vi "Append Rx Map Value to String.vi"(10 "value":T1, 11 "initial string":string) -> (3 "resulting string":string)   [LabVIEW 2020]
uses:
  Git/niveristand-ballard-milStd1553-custom-device/Source/Custom Device Support/Engine/Implementation/Rx Execution Unit/Message Map Value.ctl
  Git/niveristand-ballard-milStd1553-custom-device/Source/Custom Device Support/Shared/Message Definition.ctl
  Git/niveristand-ballard-milStd1553-custom-device/Source/Custom Device Support/Shared/Message Type.ctl
  Git/niveristand-ballard-milStd1553-custom-device/Source/Custom Device Support/Shared/Terminal Endpoint.ctl
  Git/niveristand-ballard-milStd1553-custom-device/Source/Custom Device Support/Shared/Address.ctl
  Git/niveristand-ballard-milStd1553-custom-device/Source/Custom Device Support/Shared/Parameter Definition.ctl
  Git/niveristand-ballard-milStd1553-custom-device/Source/Custom Device Support/Engine/Implementation/Rx Execution Unit/Rx Execution Unit.lvclass
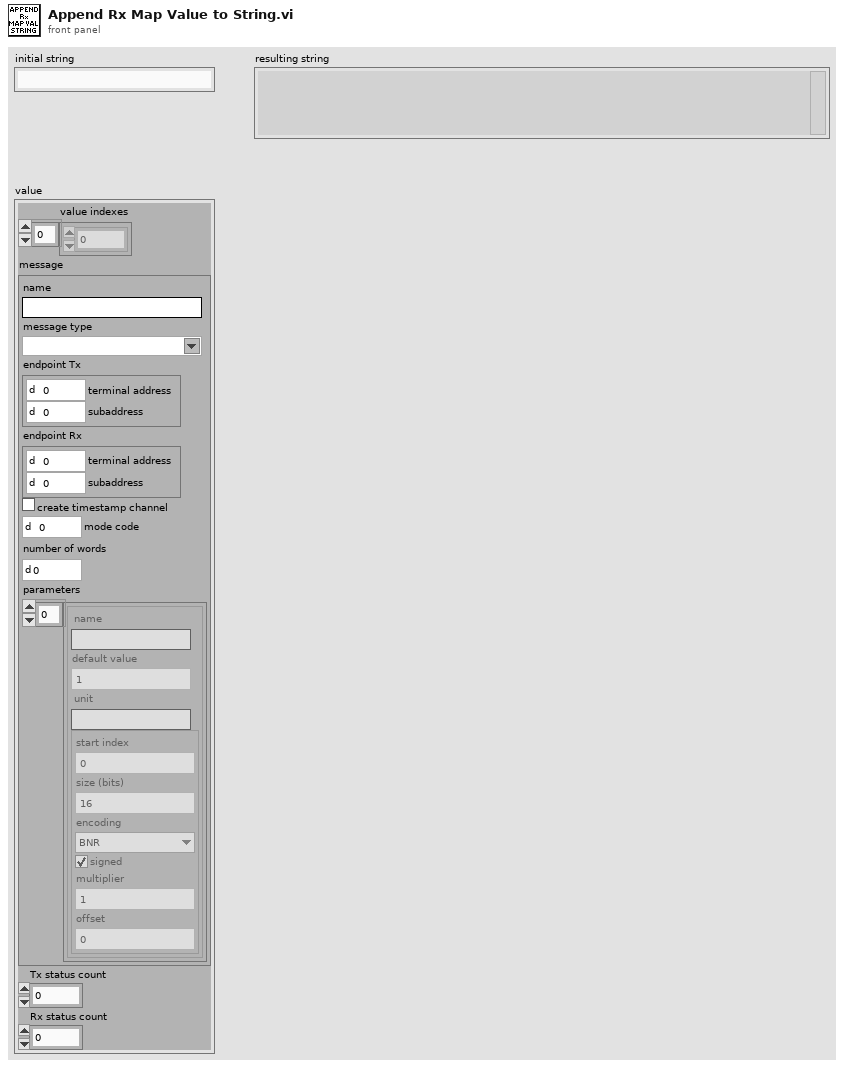
[diagram p1: front panel]
types:
  T1 = typedef "Ballard MIL-STD-1553 Engine.lvlib/Implementation.lvlib/Rx Execution Unit.lvclass/Message Map Value.ctl" = cluster{"value indexes":i32[], "message":T2, "Tx status count":i32, "Rx status count":i32}
  T2 = typedef "Message Definition.ctl" = cluster{"name":string, "message type":T3, "endpoint Tx":T4, "endpoint Rx":T4, "create timestamp channel":bool, "mode code":u16, "number of words":u16, "parameters":cluster{"name":string, "default value":dbl, "unit":string, "parameter definition":T6}[]}
  T3 = typedef "Message Type.ctl" = string
  T4 = typedef "Terminal Endpoint.ctl" = cluster{"terminal address":T5, "subaddress":T5}
  T5 = typedef "Address.ctl" = u16
  T6 = typedef "Parameter Definition.ctl" = cluster{"start index":i32, "size (bits)":i32, "encoding":enum16{"BNR", "BCD", "Discrete"}, "signed":bool, "multiplier":dbl, "offset":dbl}
  T7 = cluster{"name":string, "default value":dbl, "unit":string, "parameter definition":T6}[]
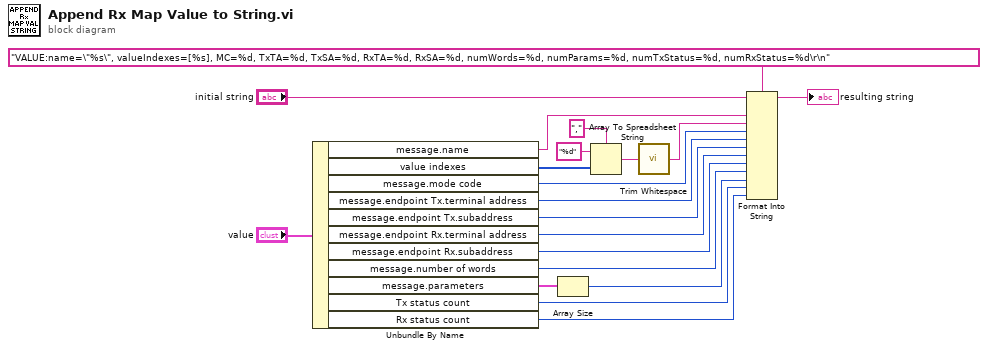
[diagram p0: block diagram]
diagram:
  n1 = Unbundle By Name("value") -> ("message.name"=w17:string, "value indexes"=w5:i32[], "message.mode code"=w8:u16, "message.endpoint Tx.terminal address"=w9:T5, "message.endpoint Tx.subaddress"=w10:T5, "message.endpoint Rx.terminal address"=w11:T5, "message.endpoint Rx.subaddress"=w12:T5, "message.number of words"=w13:u16, "message.parameters"=w4:T7, "Tx status count"=w15:i32, "Rx status count"=w16:i32)
  n2 = Array Size(array=w4) -> (size(s)=w14:i32)
  n3 = Array To Spreadsheet String(delimiter (Tab)=",", array=w5, 3:"%d" ("format string")) -> (spreadsheet string=w2:string)
  n4 = call <vilib>:"Trim Whitespace.vi"("string"=w2) -> ("trimmed string"=w1:string)  [unwired: 1 in]
  n5 = Format Into String(format string="VALUE:name=\"%s\", valueIndexes=[%s], MC=%d, TxTA=%d, TxSA=%d, RxTA=%d, RxSA=%d, numWords=%d, numParams=%d, numTxStatus=%d, numRxStatus=%d\r\n", initial string="initial string", w17, w1, w8, w9, w10, w11, w12, w13, w14, w15, w16) -> (resulting string=→"resulting string":string)  [unwired: 1 in, 1 out]
